vi "Scatter1003.vi"   [LabVIEW 2013]
uses:
  <vilib>/Heliosphere Research LLC/Advanced Plotting Toolkit/api_plotting/ScatterProperties.ctl
  <vilib>/Heliosphere Research LLC/Advanced Plotting Toolkit/properties/Marker.ctl
  <vilib>/Heliosphere Research LLC/Advanced Plotting Toolkit/properties/Marker_Style.ctl
  <vilib>/Heliosphere Research LLC/Advanced Plotting Toolkit/typedefs/PlotColor.ctl
  <vilib>/Heliosphere Research LLC/Advanced Plotting Toolkit/properties/Line.ctl
  <vilib>/Heliosphere Research LLC/Advanced Plotting Toolkit/properties/Line_Style.ctl
  <vilib>/Heliosphere Research LLC/Advanced Plotting Toolkit/properties/Colormap.ctl
  <vilib>/Heliosphere Research LLC/Advanced Plotting Toolkit/properties/Colormap_Map.ctl
  <vilib>/Heliosphere Research LLC/Advanced Plotting Toolkit/properties/Colormap_Scaling.ctl
  <vilib>/Heliosphere Research LLC/Advanced Plotting Toolkit/properties/Display.ctl
  <vilib>/Heliosphere Research LLC/Advanced Plotting Toolkit/Advanced Plotting Toolkit.lvlib
types:
  T1 = typedef "Advanced Plotting Toolkit.lvlib/Marker_Style.ctl" = enum16{"Automatic", "Circle", "Square", "Triangle", "Diamond", "Star", "Invisible"}
  T2 = typedef "Advanced Plotting Toolkit.lvlib/ScatterProperties.ctl" = cluster{"Marker":T3, "Line":T5, "Colormap":T7, "Display":T10}
  T3 = typedef "Advanced Plotting Toolkit.lvlib/Marker.ctl" = cluster{"Style":T1, "Color":T4, "Size":dbl}
  T4 = typedef "Advanced Plotting Toolkit.lvlib/PlotColor.ctl" = u32
  T5 = typedef "Advanced Plotting Toolkit.lvlib/Line.ctl" = cluster{"Style":T6, "Color":T4, "Width":sgl}
  T6 = typedef "Advanced Plotting Toolkit.lvlib/Line_Style.ctl" = enum16{"Automatic", "Solid", "Dashed", "Dotted", "Dash-dot", "Invisible"}
  T7 = typedef "Advanced Plotting Toolkit.lvlib/Colormap.ctl" = cluster{"Map":T8, "Value Min":dbl, "Value Max":dbl, "Scaling":T9, "Reverse":bool}
  T8 = typedef "Advanced Plotting Toolkit.lvlib/Colormap_Map.ctl" = enum16{"Automatic", "Rainbow", "Hot and Cold", "White-Black", "White-Blue", "White-Green", "White-Red", "Fire", "Water", "Earth", "Air", "Pastel", "Banded", "Stepped"}
  T9 = typedef "Advanced Plotting Toolkit.lvlib/Colormap_Scaling.ctl" = enum16{"Default"}
  T10 = typedef "Advanced Plotting Toolkit.lvlib/Display.ctl" = cluster{"Alpha":dbl, "Z Order":dbl}
  T11 = typedef "Advanced Plotting Toolkit.lvlib/PlotID.ctl" = i32
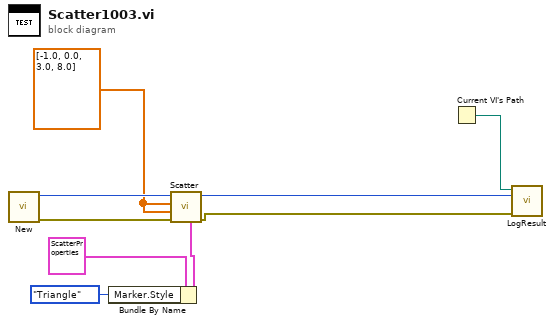
[diagram p0: block diagram]
diagram:
  w4 = dbl[] [-1.0, 0.0, 3.0, 8.0] ("X Data")
  n1 = call <vilib>:"New.vi"() -> ("error out"=w7:errorcluster, "Plot ID"=w8:T11)  [unwired: 10 in]
  n2 = Bundle By Name(cluster=T2 {"Marker"={"Style"=enum."Automatic", "Color"=2147483647, "Size"=nan}, "Line"={"Style"=enum."Automatic", "Color"=2147483647, "Width"=nan}, "Colormap"={"Map"=enum."Automatic", "Value Min"=nan, "Value Max"=nan, "Scaling"=enum."Default", "Reverse"=FALSE}, "Display"={"Alpha"=nan, "Z Order"=nan}} ("Scatter Properties"), "Marker.Style"=Marker_Style."Triangle") -> (w2:T2)
  n3 = call <vilib>:"Scatter.vi"("Properties"=w2, "error in (no error)"=w7, "Y Data"=w4, "X Data"=w4, "Plot ID"=w8) -> ("error out"=w5:errorcluster, "Plot ID Out"=w6:T11)  [unwired: 5 in]
  n4 = Current VI's Path() -> (path=w9:path)
  n5 = call "LogResult.vi"("Test Result"=w5, "Test Artifact"=w6, "VI Path"=w9) -> ()  [unwired: 9 in]
